vi "MQTT_Subscribe.vi"(8 "error in (no error)":errorcluster, 9 "Message ID":u16=10 format="%x", 10 "Subscription Info Array":cluster{"Topic":string, "QoS":T2}[](array[cluster])=[{"Topic"="a/b", "QoS"=enum."At least once"}], 11 "SSL_Connection":T1) -> (0 "error out":errorcluster, 3 "SSL_Connection 2":T1)   [LabVIEW 2015, in "MQTT_Functions.lvlib"]
doc: "This VI subscribes the client to a selected topic. The client now can read published messages for the topic. \n\n© 2015 - daq.io, LLC - Peter Adelhardt"
uses:
  LVMQTT/MQTT_Functions.lvlib
  LVMQTT/Controls/QoS.ctl
  Controls/SSL_Connection.ctl
  Controls/MessageType.ctl
  AWS_IoT.lvlib
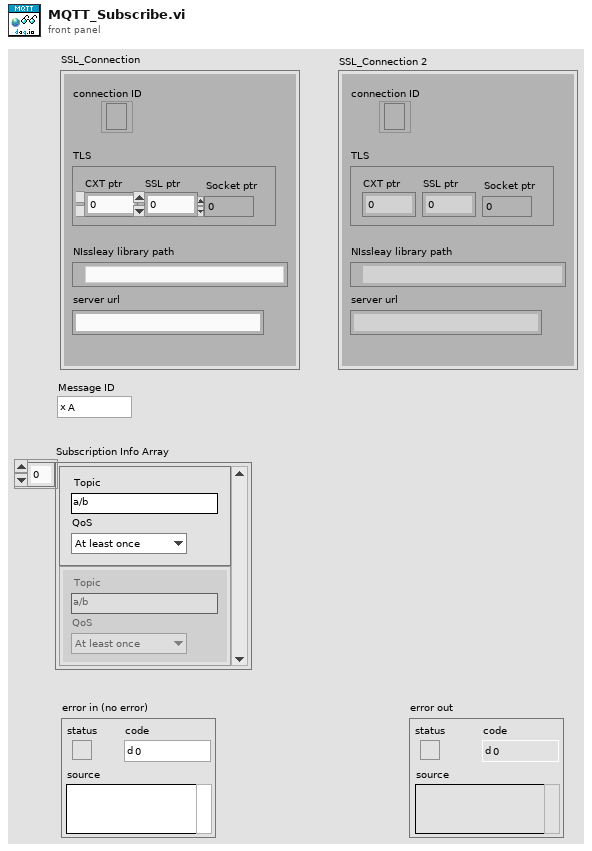
[diagram p1: front panel]
types:
  T1 = typedef "AWS_IoT.lvlib/SSL_Connection.ctl" = cluster{"connection ID":refnum<k5>, "TLS":cluster{"CXT ptr":i32, "SSL ptr":i32, "Socket ptr":i32}, "NIssleay library path":path, "server url":string}
  T2 = typedef "MQTT_Functions.lvlib/QoS.ctl" = enum8{"At most once", "At least once", "Exactly once", "Reserved"}
  T3 = typedef "MessageType.ctl" = enum32{"Reserved", "CONNECT", "CONNACK", "PUBLISH", "PUBACK", "PUBREC", "PUBREL", "PUBCOMP", "SUBSCRIBE", "SUBACK", "UNSUBSCRIBE", "UNSUBACK", "PINGREQ", "PINGRESP", "DISCONNECT", "Reserved2"}
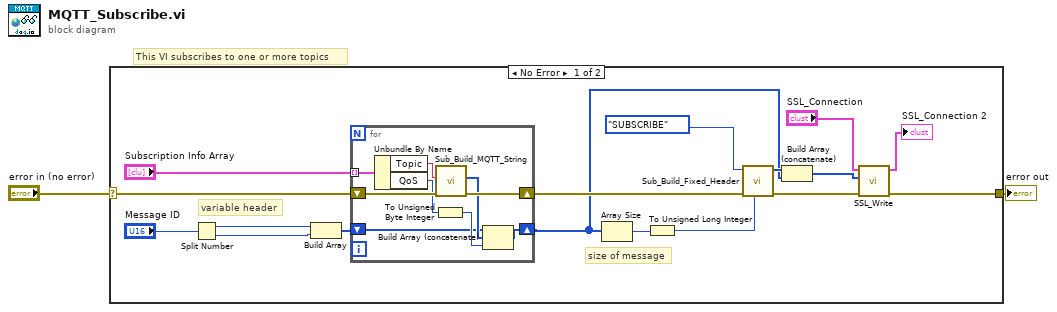
[diagram p0: block diagram]
diagram:
  # "This VI subscribes to one or more topics"
  n1 = case shown="No Error" "error in (no error)" {
    selector: "error in (no error)" -> [w13 w29]
    tunnel: [w7 w29] -> w1
    frame No Error {
      # "variable header"
      # "size of message"
      n2 = Split Number(x="Message ID") -> (hi(x)=w16:u8, lo(x)=w15:u8)
      n3 = Build Array(w16, w15) -> (w11:u8[])
      n4 = for {
        tunnel: "Subscription Info Array" -> [w28] mode=indexing
        shift-right: [w25] -> w10
        shift-left: w13 -> [w26]
        shift-right: [w21] -> w6
        shift-left: w11 -> [w20]
        n5 = Unbundle By Name(w28) -> ("Topic"=w27:string, "QoS"=w24:T2)
        n6 = To Unsigned Byte Integer(number=w24) -> (unsigned 8bit integer=w22:u8)
        n7 = call "Sub_Build_MQTT_String.vi"("error in (no error)"=w26, "String to be encoded"=w27) -> ("error out"=w25:errorcluster, "UTF8 Byte Array"=w23:u8[])  [unwired: 8 in]
        n8 = Build Array (concatenate)(w20, w23, w22) -> (w21:u8[])
      }
      n9 = Array Size(array=w6) -> (size(s)=w18:i32)
      n10 = To Unsigned Long Integer(number=w18) -> (unsigned 32bit integer=w19:u32)
      n11 = call "Sub_Build_Fixed_Header.vi"("Remaining Length"=w19, "error in (no error)"=w10, "MessageType"=MessageType."SUBSCRIBE") -> ("error out"=w8:errorcluster, "Fixed Header"=w17:u8[])  [unwired: 7 in]
      n12 = Build Array (concatenate)(w17, w6) -> (w9:u8[])
      n13 = call "SSL_Write.vi"("error in (no error)"=w8, "data in"=w9, "SSL_Connection"="SSL_Connection") -> ("error out"=w7:errorcluster, "SSL_Connection"=→"SSL_Connection 2":T1)  [unwired: 7 in]
    }
    frame Error {
    }
  }
  "error out" <- w1
